vi "Line Garage.vi"() -> ()   [LabVIEW 2017]
uses:
  <vilib>/Instr/_visa.llb/VISA Configure Serial Port (Instr).vi
  <vilib>/Utility/inputDevices.llb/keyboardAcquire.vi
panel:
  in  "Tab Control":T1(tab)
  in  "COM PORT":refnum<visa-resource-name>
  in  "Cancel Button":bool
  in  "increment":dbl
  in  "TURBINE":dbl
  out "Waveform Chart":cluster{i32, i32}(graph)
  out "RIGHT RPM":dbl
  out "LEFT RPM":dbl
  in  "RPM":bool
  out "Right Power":dbl
  out "Left Power":dbl
  out "Monitor":string
  in  "Right Motor":dbl
  in  "Left Motor":dbl
  out "Right Meter":dbl(knob) scale=-1000.0..1000.0
  out "Left Meter":dbl(knob) scale=-1000.0..1000.0
  out "RPM Graph":cluster{i32, i32}(graph)
  in  "Update":bool
  out "Right Count":dbl
  out "Left Count":dbl
  out "Sen 15":dbl
  out "Sensor 15":dbl(slide) scale=0.0..4095.0
  out "Sen 14":dbl
  out "Sensor 14":dbl(slide) scale=0.0..4095.0
  out "Sen 12":dbl
  out "Sen 11":dbl
  out "Sen 10":dbl
  out "Sen 9":dbl
  out "Sen 8":dbl
  out "Sen 7":dbl
  out "Sen 6":dbl
  out "Sen 5":dbl
  out "Sen 4":dbl
  out "Sen 3":dbl
  out "Sen 2":dbl
  out "Sen 1":dbl
  out "Sen 0":dbl
  out "Sensor 12":dbl(slide) scale=0.0..4095.0
  out "Sensor 10":dbl(slide) scale=0.0..4095.0
  out "Sensor 9":dbl(slide) scale=0.0..4095.0
  out "Sensor 8":dbl(slide) scale=0.0..4095.0
  out "Sensor 7":dbl(slide) scale=0.0..4095.0
  out "Sensor 6":dbl(slide) scale=0.0..4095.0
  out "Sensor 5":dbl(slide) scale=0.0..4095.0
  out "Sensor 4":dbl(slide) scale=0.0..4095.0
  out "Sensor 3":dbl(slide) scale=0.0..4095.0
  out "Sensor 2":dbl(slide) scale=0.0..4095.0
  out "Sensor 1":dbl(slide) scale=0.0..4095.0
  out "Sensor 0":dbl(slide) scale=0.0..4095.0
  out "Sensor 11":dbl(slide) scale=0.0..4095.0
  in  "Update Sensors":bool
  out "Sensor 13":dbl(slide) scale=0.0..4095.0
  out "Sen 13":dbl
  in  "Read Calibration":bool
  in  "Save Calibration EEPROM":bool
  out "Max 14":dbl
  out "Min 14":dbl
  out "SenM 14":dbl
  out "SensorM 14":dbl(slide) scale=0.0..1000.0
  out "Max 13":dbl
  out "Min 13":dbl
  out "SenM 13":dbl
  out "SensorM 13":dbl(slide) scale=0.0..1000.0
  out "Max 12":dbl
  out "Max 11":dbl
  out "Max 10":dbl
  out "Max 9":dbl
  out "Max 8":dbl
  out "Max 7":dbl
  out "Max 6":dbl
  out "Max 5":dbl
  out "Max 4":dbl
  out "Max 3":dbl
  out "Max 2":dbl
  out "Max 1":dbl
  out "Max 0":dbl
  out "Min 12":dbl
  out "Min 11":dbl
  out "Min 10":dbl
  out "Min 9":dbl
  out "Min 8":dbl
  out "Min 7":dbl
  out "Min 6":dbl
  out "Min 5":dbl
  out "Min 4":dbl
  out "Min 3":dbl
  out "Min 2":dbl
  out "Min 1":dbl
  out "Min 0":dbl
  out "SenM 12":dbl
  out "SenM 11":dbl
  out "SenM 10":dbl
  out "SenM 9":dbl
  out "SenM 8":dbl
  out "SenM 7":dbl
  out "SenM 6":dbl
  out "SenM 5":dbl
  out "SenM 4":dbl
  out "SenM 3":dbl
  out "SenM 2":dbl
  out "SenM 1":dbl
  out "SenM 0":dbl
  out "SensorM 12":dbl(slide) scale=0.0..1000.0
  out "SensorM 10":dbl(slide) scale=0.0..1000.0
  out "SensorM 9":dbl(slide) scale=0.0..1000.0
  out "SensorM 8":dbl(slide) scale=0.0..1000.0
  out "SensorM 7":dbl(slide) scale=0.0..1000.0
  out "SensorM 6":dbl(slide) scale=0.0..1000.0
  out "SensorM  5":dbl(slide) scale=0.0..1000.0
  out "SensorM 4":dbl(slide) scale=0.0..1000.0
  out "SensorM 3":dbl(slide) scale=0.0..1000.0
  out "SensorM 2":dbl(slide) scale=0.0..1000.0
  out "SensorM 1":dbl(slide) scale=0.0..1000.0
  out "SensorM 0":dbl(slide) scale=0.0..1000.0
  out "SensorM 11":dbl(slide) scale=0.0..1000.0
  in  "Update Sensors 2":bool
  out "SensorM 15":dbl(slide) scale=0.0..1000.0
  out "SenM 15":dbl
  out "Min 15":dbl
  out "Max 15":dbl
  out "Position":dbl
  in  "Graph":bool
  out "Position":cluster{i32, i32}(graph)
  in  "Up Turbine":bool
  in  "Read Values":bool
  in  "Read EEPROM":bool
  in  "Save EEPROM":bool
  in  "Up Max":bool
  in  "Up Min":bool
  in  "Max Rang":dbl
  in  "Min Rang":dbl
  in  "Turbine Speed":dbl
  in  "Max In_1":dbl
  in  "Max D_1":dbl
  in  "Up MainSpeed":bool
  in  "Main Speed":dbl
  in  "Up Button1":bool
  in  "Kd_1":dbl
  in  "Ki_1":dbl
  in  "sample Time_1":dbl
  in  "SetPoint_1":dbl
  in  "Kp_1":dbl
  in  "Kp_2":dbl
  in  "SetPoint_2":dbl
  in  "sample Time_2":dbl
  in  "Ki_2":dbl
  in  "Kd_2":dbl
  in  "Up Button 2":bool
  in  "Max D_2":dbl
  in  "Max In_2":dbl
  in  "Max In_3":dbl
  in  "Max D_3":dbl
  in  "Up Button 3":bool
  in  "Kd_3":dbl
  in  "Ki_3":dbl
  in  "sample Time_3":dbl
  in  "SetPoint_3":dbl
  in  "Kp_3":dbl
  # "RIGHT"
  # "Motors"
  # "LEFT"
  # "Encoders Counts"
  # "LATERAL_PID"
  # "Turbine_PID"
  # "Central"
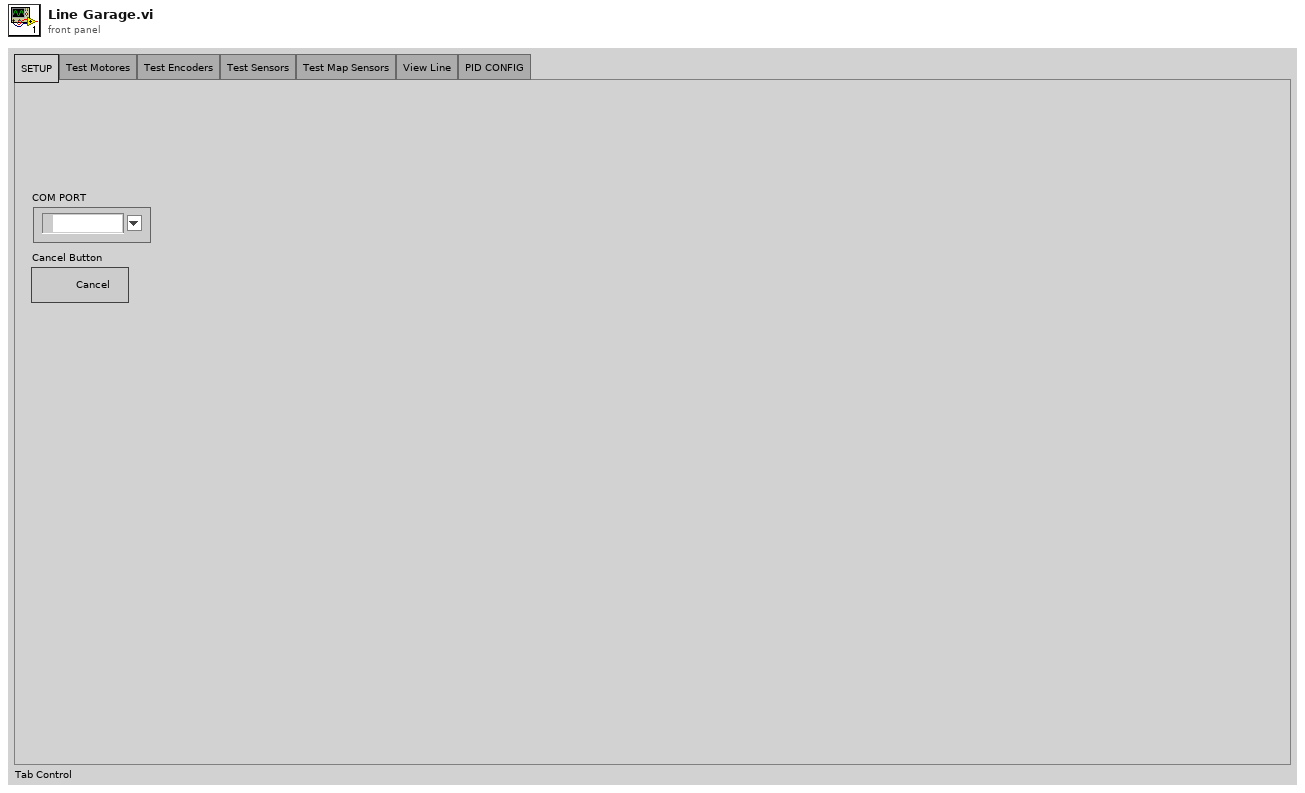
[diagram p1: front panel]
types:
  T1 = enum32{"SETUP", "Test Motores", "Test Encoders", "Test Sensors", "Test Map Sensors", "View Line", "PID CONFIG"}
  T2 = enum16{"0", "1", "2", "3", "4", "5", "6", "7", "8", "9", "A", "B", "C", "D", "E", "F", "G", "H", "I", "J", "K", "L", "M", "N", "O", "P", "Q", "R", "S", "T", "U", "V", "W", "X", "Y", "Z", "F1", "F2", "F3", "F4", "F5", "F6", "F7", "F8", "F9", "F10", "F11", "F12", "F13", "F14", "F15", "ADD", "BACK", "BACKSLASH", "CAPITAL", "COMMA", "DECIMAL", "DELETE", "DIVIDE", "DOWN", "END", "EQUALS", "ESCAPE", "GRAVE (`)", "HOME", "INSERT", "LBRACKET", "LCONTROL", "LEFT", "L ALT", "LSHIFT", "LWIN", "MINUS", "MULTIPLY", "NEXT", "NUMLOCK", "NUMPAD_0", "NUMPAD_1", "NUMPAD_2", "NUMPAD_3", "NUMPAD_4", "NUMPAD_5", "NUMPAD_6", "NUMPAD_7", "NUMPAD_8", "NUMPAD_9", "PAUSE", "PERIOD", "PRIOR (PG UP)", "RBRACKET", "RCONTROL", "RETURN", "RIGHT", "R ALT", "RSHIFT", "RWIN", "SCROLL", "SEMICOLON", "SLASH", "SPACE", "SUBTRACT", "TAB", "UP", "ENTER (num pad)", "' (quote)"}[]
  T3 = enum16{"0", "1", "2", "3", "4", "5", "6", "7", "8", "9", "A", "B", "C", "D", "E", "F", "G", "H", "I", "J", "K", "L", "M", "N", "O", "P", "Q", "R", "S", "T", "U", "V", "W", "X", "Y", "Z", "F1", "F2", "F3", "F4", "F5", "F6", "F7", "F8", "F9", "F10", "F11", "F12", "F13", "F14", "F15", "ADD", "BACK", "BACKSLASH", "CAPITAL", "COMMA", "DECIMAL", "DELETE", "DIVIDE", "DOWN", "END", "EQUALS", "ESCAPE", "GRAVE (`)", "HOME", "INSERT", "LBRACKET", "LCONTROL", "LEFT", "L ALT", "LSHIFT", "LWIN", "MINUS", "MULTIPLY", "NEXT", "NUMLOCK", "NUMPAD_0", "NUMPAD_1", "NUMPAD_2", "NUMPAD_3", "NUMPAD_4", "NUMPAD_5", "NUMPAD_6", "NUMPAD_7", "NUMPAD_8", "NUMPAD_9", "PAUSE", "PERIOD", "PRIOR (PG UP)", "RBRACKET", "RCONTROL", "RETURN", "RIGHT", "R ALT", "RSHIFT", "RWIN", "SCROLL", "SEMICOLON", "SLASH", "SPACE", "SUBTRACT", "TAB", "UP", "ENTER (num pad)", "' (quote)"}
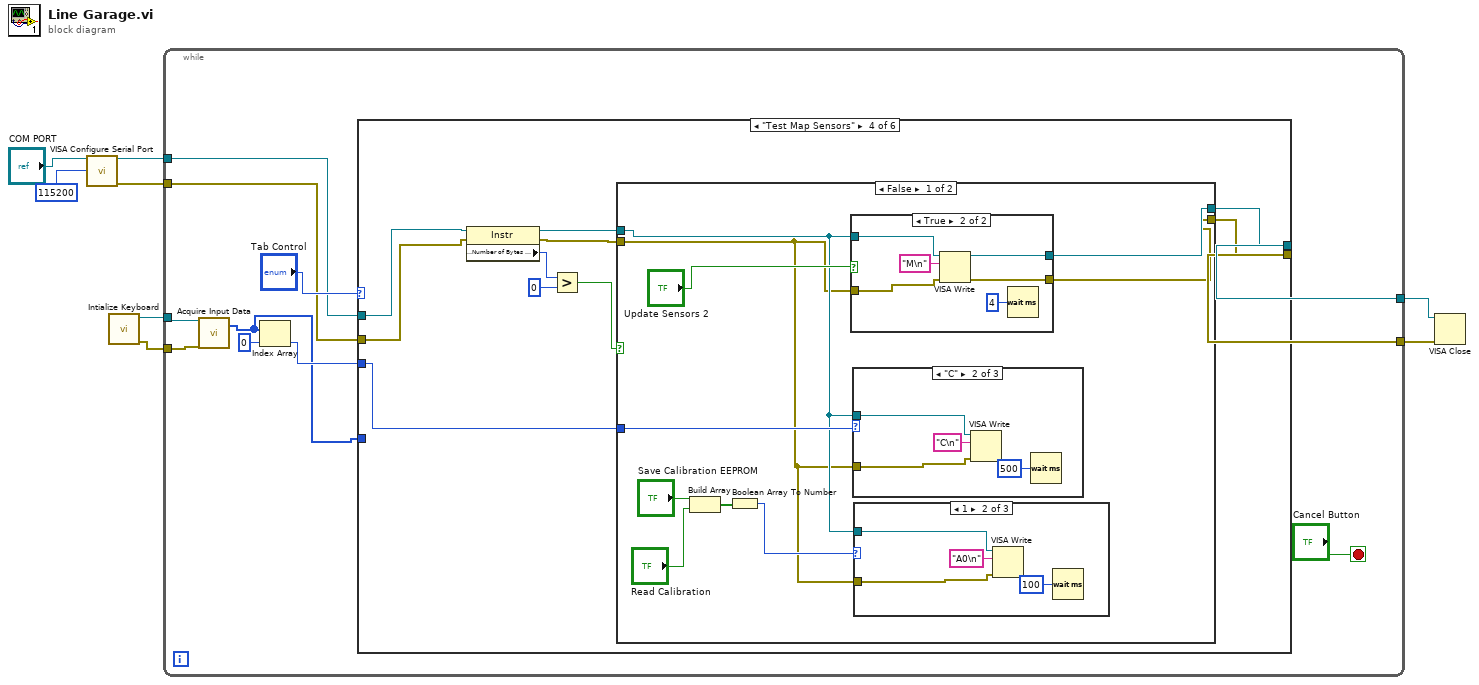
[diagram p0: block diagram]
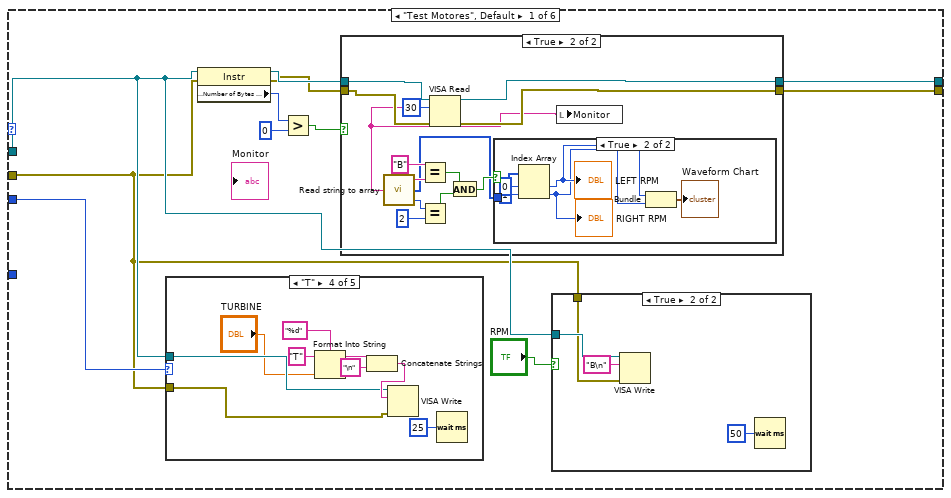
[diagram p2: hidden frame]
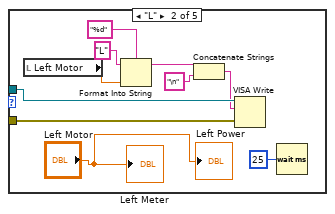
[diagram p7: hidden frame]
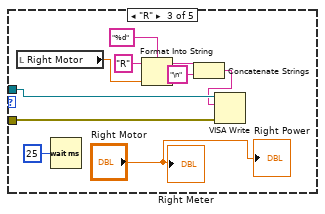
[diagram p8: hidden frame]
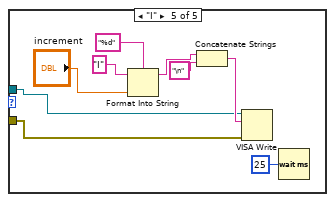
[diagram p9: hidden frame]
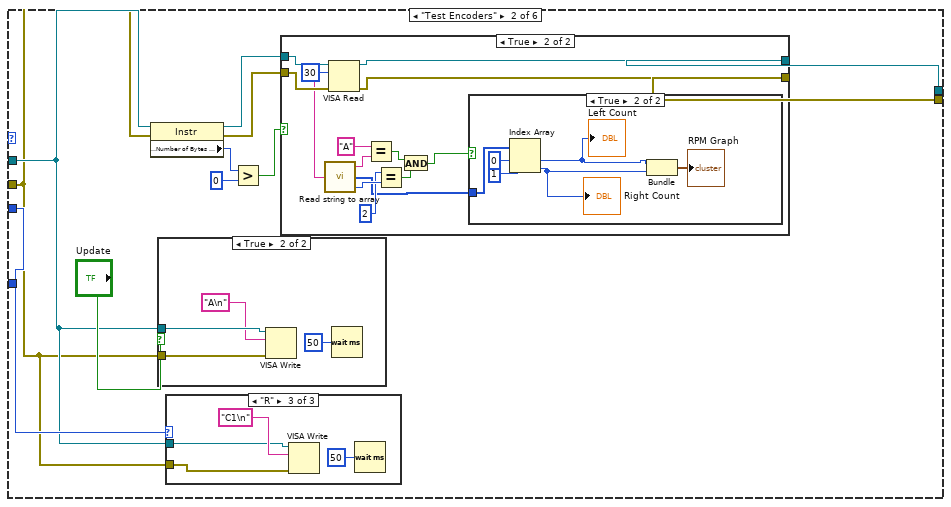
[diagram p10: hidden frame]
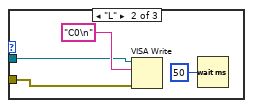
[diagram p12: hidden frame]
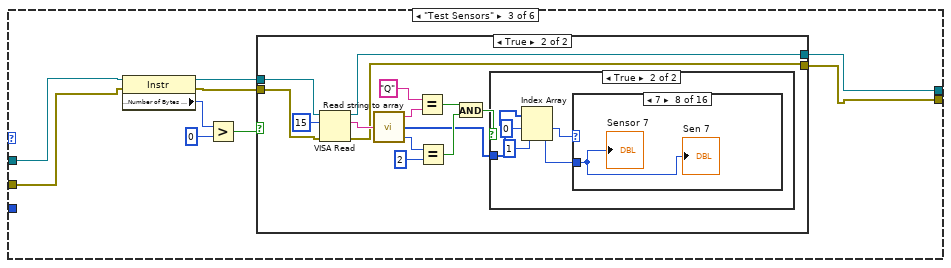
[diagram p16: hidden frame]
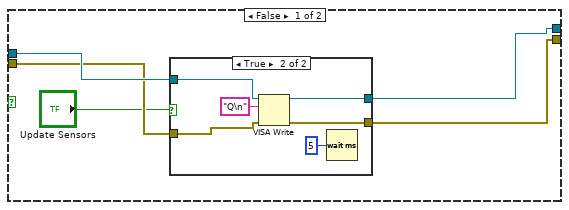
[diagram p17: hidden frame]
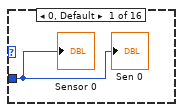
[diagram p20: hidden frame]
diagram:
  n1 = call-poly "VISA Configure Serial Port"("VISA resource name"="COM PORT", "baud rate (9600)"=u32 115200) -> ("VISA resource name out"=w4:refnum<visa-resource-name>, "error out"=w3:errorcluster)  [unwired: 12 in]
  n2 = call <vilib>:"Intialize Keyboard.vi"() -> ("error out"=w7:errorcluster, "device ID"=w8:refnum<k1>)  [unwired: 10 in]
  n3 = while {
    tunnel: w8 -> [w18]
    tunnel: w7 -> [w17]
    tunnel: w4 -> [w13]
    tunnel: w3 -> [w12]
    tunnel: [w11] -> w2
    tunnel: [w10] -> w1
    stop <- "Cancel Button" stop-if-true
    n4 = call-poly <vilib>:"Acquire Input Data.vi"("device ID"=w18, "error in (no error)"=w17) -> ("keys pressed"=w9:T2)  [unwired: 15 in, 2 out]
    n5 = Index Array(array=w9, index=0) -> (element=w14:T3)
    n6 = case shown="\"Test Map Sensors\"" "Tab Control" {
      tunnel: w14 -> [w30 w97 _ w197 _ w365]
      tunnel: w13 -> [w21 w96 w141 w204 w332 w374]
      tunnel: w12 -> [w20 w95 w140 w203 w331 w373]
      tunnel: [w25 w100 w142 w198 w324 w367] -> w11
      tunnel: [w23 w98 w143 w199 w325 w366] -> w10
      tunnel: w9 -> [_ _ _ _ _ _]
      frame "Test Motores", Default {
        n7 = case shown="\"T\"" w30 {
          tunnel: w21 -> [_ w66 w75 w78 w88]
          tunnel: w20 -> [_ w65 w74 w79 w87]
          frame "0", Default {
          }
          frame "L" {
            n8 = local read "Left Motor"() -> (w61:dbl)
            n9 = Format Into String(format string="%d", initial string="L", w61) -> (resulting string=w60:string)  [unwired: 1 in, 1 out]
            n10 = Concatenate Strings(w60, "\n" ("string")) -> (w58:string)
            n11 = VISA Write(VISA resource name=w66, write buffer=w58, error in (no error)=w65) -> ()  [unwired: 3 out]
            n12 = Wait (ms)(milliseconds to wait=u32 25) -> ()  [unwired: 1 out]
            "Left Meter" <- "Left Motor"
            "Left Power" <- "Left Motor"
          }
          frame "R" {
            n13 = local read "Right Motor"() -> (w71:dbl)
            n14 = Wait (ms)(milliseconds to wait=u32 25) -> ()  [unwired: 1 out]
            n15 = Format Into String(format string="%d", initial string="R", w71) -> (resulting string=w69:string)  [unwired: 1 in, 1 out]
            n16 = Concatenate Strings(w69, "\n" ("string")) -> (w70:string)
            n17 = VISA Write(VISA resource name=w75, write buffer=w70, error in (no error)=w74) -> ()  [unwired: 3 out]
            "Right Meter" <- "Right Motor"
            "Right Power" <- "Right Motor"
          }
          frame "T" {
            n18 = Format Into String(format string="%d", initial string="T", "TURBINE") -> (resulting string=w81:string)  [unwired: 1 in, 1 out]
            n19 = Concatenate Strings(w81, "\n" ("string")) -> (w82:string)
            n20 = VISA Write(VISA resource name=w78, write buffer=w82, error in (no error)=w79) -> ()  [unwired: 3 out]
            n21 = Wait (ms)(milliseconds to wait=u32 25) -> ()  [unwired: 1 out]
          }
          frame "I" {
            n22 = Format Into String(format string="%d", initial string="I", "increment") -> (resulting string=w91:string)  [unwired: 1 in, 1 out]
            n23 = Concatenate Strings(w91, "\n") -> (w89:string)
            n24 = VISA Write(VISA resource name=w88, write buffer=w89, error in (no error)=w87) -> ()  [unwired: 3 out]
            n25 = Wait (ms)(milliseconds to wait=u32 25) -> ()  [unwired: 1 out]
          }
        }
        n26 = property class="Instr"(reference=w21, error in=w20) -> (reference out=w26:refnum<visa-resource-name>, error out=w24:errorcluster, "Serial Settings:Number of Bytes at Serial Port"=w29:u32)
        n27 = Greater?(x=w29, y=u32 0) -> (0:w27:bool)
        n28 = case shown="True" w27 {
          tunnel: [w36 w48] -> w25
          tunnel: w26 -> [w36 w50]
          tunnel: w24 -> [w35 w49]
          tunnel: [w35 w47] -> w23
          frame False {
          }
          frame True {
            n29 = VISA Read(VISA resource name=w50, byte count=u32 30, error in (no error)=w49) -> (VISA resource name out=w48:refnum<visa-resource-name>, read buffer=w45:string, error out=w47:errorcluster)  [unwired: 1 out]
            n30 = call "Read string to array.vi"("String"=w45) -> ("size(s)"=w40:i32, "Array"=w37:i32[], "caracter"=w44:string)  [unwired: 2 in]
            n31 = Equal?(x="B", y=w44) -> (x = y?=w42:bool)
            n32 = Equal?(x=w40, y=2) -> (x = y?=w41:bool)
            n33 = And(x=w42, y=w41) -> (x .and. y?=w38:bool)
            n34 = case shown="True" w38 {
              tunnel: w37 -> [_ w56]
              frame False {
              }
              frame True {
                n35 = Index Array(array=w56, index #1=0 ("index"), index #2=1 ("index")) -> (element #1=w53:i32, element #2=w52:i32)
                "LEFT RPM" <- w53
                "RIGHT RPM" <- w52
                n36 = Bundle(w53, w52) -> (→"Waveform Chart":cluster{i32, i32})  [unwired: 1 in]
              }
            }
            n37 = local write "Monitor"(w45) -> ()
          }
        }
        n38 = case shown="True" "RPM" {
          tunnel: w21 -> [_ w34]
          tunnel: w20 -> [_ w33]
          frame False {
          }
          frame True {
            n39 = VISA Write(VISA resource name=w34, write buffer="B\n", error in (no error)=w33) -> ()  [unwired: 3 out]
            n40 = Wait (ms)(milliseconds to wait=u32 50) -> ()  [unwired: 1 out]
          }
        }
      }
      frame "Test Encoders" {
        n41 = property class="Instr"(reference=w96, error in=w95) -> (reference out=w101:refnum<visa-resource-name>, error out=w99:errorcluster, "Serial Settings:Number of Bytes at Serial Port"=w104:u32)
        n42 = case shown="True" "Update" {
          tunnel: w96 -> [_ w138]
          tunnel: w95 -> [_ w137]
          frame False {
          }
          frame True {
            n43 = VISA Write(VISA resource name=w138, write buffer="A\n", error in (no error)=w137) -> ()  [unwired: 3 out]
            n44 = Wait (ms)(milliseconds to wait=u32 50) -> ()  [unwired: 1 out]
          }
        }
        n45 = case shown="\"R\"" w97 {
          tunnel: w96 -> [_ w107 w111]
          tunnel: w95 -> [_ w106 w110]
          frame "0", Default {
          }
          frame "L" {
            n46 = VISA Write(VISA resource name=w107, write buffer="C0\n", error in (no error)=w106) -> ()  [unwired: 3 out]
            n47 = Wait (ms)(milliseconds to wait=u32 50) -> ()  [unwired: 1 out]
          }
          frame "R" {
            n48 = VISA Write(VISA resource name=w111, write buffer="C1\n", error in (no error)=w110) -> ()  [unwired: 3 out]
            n49 = Wait (ms)(milliseconds to wait=u32 50) -> ()  [unwired: 1 out]
          }
        }
        n50 = Greater?(x=w104, y=u32 0) -> (0:w102:bool)
        n51 = case shown="True" w102 {
          tunnel: [w115 w126] -> w100
          tunnel: w101 -> [w115 w129]
          tunnel: [w114 w125] -> w98
          tunnel: w99 -> [w114 w128]
          frame False {
          }
          frame True {
            n52 = VISA Read(VISA resource name=w129, byte count=u32 30, error in (no error)=w128) -> (VISA resource name out=w126:refnum<visa-resource-name>, read buffer=w124:string, error out=w125:errorcluster)  [unwired: 1 out]
            n53 = call "Read string to array.vi"("String"=w124) -> ("size(s)"=w120:i32, "Array"=w116:i32[], "caracter"=w123:string)  [unwired: 2 in]
            n54 = Equal?(x="A", y=w123) -> (x = y?=w121:bool)
            n55 = Equal?(x=2, y=w120) -> (x = y?=w118:bool)
            n56 = And(x=w121, y=w118) -> (x .and. y?=w117:bool)
            n57 = case shown="True" w117 {
              tunnel: w116 -> [_ w135]
              frame False {
              }
              frame True {
                n58 = Index Array(array=w135, index #1=0 ("index"), index #2=1 ("index")) -> (element #1=w132:i32, element #2=w130:i32)
                "Right Count" <- w130
                "Left Count" <- w132
                n59 = Bundle(w132, w130) -> (→"RPM Graph":cluster{i32, i32})  [unwired: 1 in]
              }
            }
          }
        }
      }
      frame "Test Sensors" {
        n60 = property class="Instr"(reference=w141, error in=w140) -> (reference out=w145:refnum<visa-resource-name>, error out=w144:errorcluster, "Serial Settings:Number of Bytes at Serial Port"=w148:u32)
        n61 = Greater?(x=w148, y=u32 0) -> (0:w146:bool)
        n62 = case shown="True" w146 {
          tunnel: w145 -> [w153 w175]
          tunnel: w144 -> [w152 w174]
          tunnel: [w150 w163] -> w142
          tunnel: [w149 w162] -> w143
          frame False {
            n63 = case shown="True" "Update Sensors" {
              tunnel: w153 -> [w155 w160]
              tunnel: w152 -> [w154 w159]
              tunnel: [w155 w158] -> w150
              tunnel: [w154 w157] -> w149
              frame False {
              }
              frame True {
                n64 = VISA Write(VISA resource name=w160, write buffer="Q\n", error in (no error)=w159) -> (VISA resource name out=w158:refnum<visa-resource-name>, error out=w157:errorcluster)  [unwired: 1 out]
                n65 = Wait (ms)(milliseconds to wait=u32 5) -> ()  [unwired: 1 out]
              }
            }
          }
          frame True {
            n66 = VISA Read(VISA resource name=w175, byte count=u32 15, error in (no error)=w174) -> (VISA resource name out=w163:refnum<visa-resource-name>, read buffer=w172:string, error out=w162:errorcluster)  [unwired: 1 out]
            n67 = call "Read string to array.vi"("String"=w172) -> ("size(s)"=w169:i32, "Array"=w164:i32[], "caracter"=w171:string)  [unwired: 2 in]
            n68 = Equal?(x="Q", y=w171) -> (x = y?=w167:bool)
            n69 = Equal?(x=w169, y=2) -> (x = y?=w166:bool)
            n70 = And(x=w167, y=w166) -> (x .and. y?=w165:bool)
            n71 = case shown="True" w165 {
              tunnel: w164 -> [_ w180]
              frame False {
              }
              frame True {
                n72 = Index Array(array=w180, index #1=0 ("index"), index #2=1 ("index")) -> (element #1=w177:i32, element #2=w176:i32)
                n73 = case shown="7" w177 {
                  tunnel: w176 -> [w181 w182 w183 w184 w185 w186 w187 w188 w189 w190 w191 w192 w193 w194 w195 w196]
                  frame 0, Default {
                    "Sensor 0" <- w181
                    "Sen 0" <- w181
                  }
                  frame 1 {
                    "Sensor 1" <- w182
                    "Sen 1" <- w182
                  }
                  frame 2 {
                    "Sen 2" <- w183
                    "Sensor 2" <- w183
                  }
                  frame 3 {
                    "Sensor 3" <- w184
                    "Sen 3" <- w184
                  }
                  frame 4 {
                    "Sensor 4" <- w185
                    "Sen 4" <- w185
                  }
                  frame 5 {
                    "Sen 5" <- w186
                    "Sensor 5" <- w186
                  }
                  frame 6 {
                    "Sensor 6" <- w187
                    "Sen 6" <- w187
                  }
                  frame 7 {
                    "Sensor 7" <- w188
                    "Sen 7" <- w188
                  }
                  frame 8 {
                    "Sensor 8" <- w189
                    "Sen 8" <- w189
                  }
                  frame 9 {
                    "Sensor 9" <- w190
                    "Sen 9" <- w190
                  }
                  frame 10 {
                    "Sensor 10" <- w191
                    "Sen 10" <- w191
                  }
                  frame 11 {
                    "Sensor 11" <- w192
                    "Sen 11" <- w192
                  }
                  frame 12 {
                    "Sen 12" <- w193
                    "Sensor 12" <- w193
                  }
                  frame 13 {
                    "Sen 13" <- w194
                    "Sensor 13" <- w194
                  }
                  frame 14 {
                    "Sensor 14" <- w195
                    "Sen 14" <- w195
                  }
                  frame 15 {
                    "Sensor 15" <- w196
                    "Sen 15" <- w196
                  }
                }
              }
            }
          }
        }
      }
      frame "Test Map Sensors" {
        n74 = property class="Instr"(reference=w204, error in=w203) -> (reference out=w201:refnum<visa-resource-name>, error out=w200:errorcluster, "Serial Settings:Number of Bytes at Serial Port"=w206:u32)
        n75 = Greater?(x=w206, y=u32 0) -> (0:w202:bool)
        n76 = case shown="False" w202 {
          tunnel: w201 -> [w208 w259]
          tunnel: w200 -> [w207 w258]
          tunnel: [w215 w253] -> w198
          tunnel: [w214 w252] -> w199
          tunnel: w197 -> [w213 _]
          frame False {
            n77 = Build Array("Save Calibration EEPROM", "Read Calibration") -> (w210:bool[])
            n78 = Boolean Array To Number(Boolean array=w210) -> (number=w209:u32)
            n79 = case shown="True" "Update Sensors 2" {
              tunnel: w208 -> [w234 w239]
              tunnel: w207 -> [w233 w238]
              tunnel: [w234 w237] -> w215
              tunnel: [w233 w236] -> w214
              frame False {
              }
              frame True {
                n80 = VISA Write(VISA resource name=w239, write buffer="M\n", error in (no error)=w238) -> (VISA resource name out=w237:refnum<visa-resource-name>, error out=w236:errorcluster)  [unwired: 1 out]
                n81 = Wait (ms)(milliseconds to wait=u32 4) -> ()  [unwired: 1 out]
              }
            }
            n82 = case shown="\"C\"" w213 {
              tunnel: w208 -> [_ w227 w230]
              tunnel: w207 -> [_ w226 w229]
              frame "0", Default {
              }
              frame "C" {
                n83 = VISA Write(VISA resource name=w227, write buffer="C\n", error in (no error)=w226) -> ()  [unwired: 3 out]
                n84 = Wait (ms)(milliseconds to wait=u32 500) -> ()  [unwired: 1 out]
              }
              frame "G" {
                n85 = VISA Write(VISA resource name=w230, write buffer="G\n", error in (no error)=w229) -> ()  [unwired: 3 out]
                n86 = Wait (ms)(milliseconds to wait=u32 500) -> ()  [unwired: 1 out]
              }
            }
            n87 = case shown="1" w209 {
              tunnel: w208 -> [_ w218 w221]
              tunnel: w207 -> [_ w217 w222]
              frame 0, Default {
              }
              frame 1 {
                n88 = VISA Write(VISA resource name=w218, write buffer="A0\n", error in (no error)=w217) -> ()  [unwired: 3 out]
                n89 = Wait (ms)(milliseconds to wait=u32 100) -> ()  [unwired: 1 out]
              }
              frame 2 {
                n90 = VISA Write(VISA resource name=w221, write buffer="B0\n", error in (no error)=w222) -> ()  [unwired: 3 out]
                n91 = Wait (ms)(milliseconds to wait=u32 100) -> ()  [unwired: 1 out]
              }
            }
          }
          frame True {
            n92 = VISA Read(VISA resource name=w259, byte count=u32 15, error in (no error)=w258) -> (VISA resource name out=w253:refnum<visa-resource-name>, read buffer=w247:string, error out=w252:errorcluster)  [unwired: 1 out]
            n93 = call "Read string to array.vi"("String"=w247) -> ("size(s)"=w251:i32, "Array"=w242:i32[], "caracter"=w241:string)  [unwired: 2 in]
            n94 = Equal?(x=w241, y="U") -> (x = y?=w248:bool)
            n95 = Equal?(x="M", y=w241) -> (x = y?=w255:bool)
            n96 = Equal?(x=w251, y=2) -> (x = y?=w245:bool)
            n97 = And(x=w248, y=w245) -> (x .and. y?=w249:bool)
            n98 = case shown="True" w249 {
              tunnel: w242 -> [_ w286]
              frame False {
              }
              frame True {
                n99 = Index Array(array=w286, index #1=0 ("index"), index #2=1 ("index")) -> (element #1=w283:i32, element #2=w282:i32)
                n100 = case shown="15" w283 {
                  tunnel: w282 -> [w287 w288 w289 w290 w291 w292 w293 w294 w295 w296 w297 w298 w299 w300 w301 w302]
                  frame 0, Default {
                    "Max 0" <- w287
                  }
                  frame 1 {
                    "Max 1" <- w288
                  }
                  frame 2 {
                    "Max 2" <- w289
                  }
                  frame 3 {
                    "Max 3" <- w290
                  }
                  frame 4 {
                    "Max 4" <- w291
                  }
                  frame 5 {
                    "Max 5" <- w292
                  }
                  frame 6 {
                    "Max 6" <- w293
                  }
                  frame 7 {
                    "Max 7" <- w294
                  }
                  frame 8 {
                    "Max 8" <- w295
                  }
                  frame 9 {
                    "Max 9" <- w296
                  }
                  frame 10 {
                    "Max 10" <- w297
                  }
                  frame 11 {
                    "Max 11" <- w298
                  }
                  frame 12 {
                    "Max 12" <- w299
                  }
                  frame 13 {
                    "Max 13" <- w300
                  }
                  frame 14 {
                    "Max 14" <- w301
                  }
                  frame 15 {
                    "Max 15" <- w302
                  }
                }
              }
            }
            n101 = And(x=w255, y=w245) -> (x .and. y?=w254:bool)
            n102 = case shown="True" w254 {
              tunnel: w242 -> [_ w307]
              frame False {
              }
              frame True {
                n103 = Index Array(array=w307, index #1=0 ("index"), index #2=1 ("index")) -> (element #1=w304:i32, element #2=w303:i32)
                n104 = case shown="15" w304 {
                  tunnel: w303 -> [w308 w309 w310 w311 w312 w313 w314 w315 w316 w317 w318 w319 w320 w321 w322 w323]
                  frame 0, Default {
                    "SenM 0" <- w308
                    "SensorM 0" <- w308
                  }
                  frame 1 {
                    "SenM 1" <- w309
                    "SensorM 1" <- w309
                  }
                  frame 2 {
                    "SensorM 2" <- w310
                    "SenM 2" <- w310
                  }
                  frame 3 {
                    "SensorM 3" <- w311
                    "SenM 3" <- w311
                  }
                  frame 4 {
                    "SensorM 4" <- w312
                    "SenM 4" <- w312
                  }
                  frame 5 {
                    "SensorM  5" <- w313
                    "SenM 5" <- w313
                  }
                  frame 6 {
                    "SensorM 6" <- w314
                    "SenM 6" <- w314
                  }
                  frame 7 {
                    "SensorM 7" <- w315
                    "SenM 7" <- w315
                  }
                  frame 8 {
                    "SensorM 8" <- w316
                    "SenM 8" <- w316
                  }
                  frame 9 {
                    "SenM 9" <- w317
                    "SensorM 9" <- w317
                  }
                  frame 10 {
                    "SensorM 10" <- w318
                    "SenM 10" <- w318
                  }
                  frame 11 {
                    "SensorM 11" <- w319
                    "SenM 11" <- w319
                  }
                  frame 12 {
                    "SenM 12" <- w320
                    "SensorM 12" <- w320
                  }
                  frame 13 {
                    "SenM 13" <- w321
                    "SensorM 13" <- w321
                  }
                  frame 14 {
                    "SensorM 14" <- w322
                    "SenM 14" <- w322
                  }
                  frame 15 {
                    "SensorM 15" <- w323
                    "SenM 15" <- w323
                  }
                }
              }
            }
            n105 = Equal?(x=w241, y="L") -> (x = y?=w244:bool)
            n106 = And(x=w245, y=w244) -> (x .and. y?=w243:bool)
            n107 = case shown="True" w243 {
              tunnel: w242 -> [_ w265]
              frame False {
              }
              frame True {
                n108 = Index Array(array=w265, index #1=0 ("index"), index #2=1 ("index")) -> (element #1=w262:i32, element #2=w261:i32)
                n109 = case shown="15" w262 {
                  tunnel: w261 -> [w266 w267 w268 w269 w270 w271 w272 w273 w274 w275 w276 w277 w278 w279 w280 w281]
                  frame 0, Default {
                    "Min 0" <- w266
                  }
                  frame 1 {
                    "Min 1" <- w267
                  }
                  frame 2 {
                    "Min 2" <- w268
                  }
                  frame 3 {
                    "Min 3" <- w269
                  }
                  frame 4 {
                    "Min 4" <- w270
                  }
                  frame 5 {
                    "Min 5" <- w271
                  }
                  frame 6 {
                    "Min 6" <- w272
                  }
                  frame 7 {
                    "Min 7" <- w273
                  }
                  frame 8 {
                    "Min 8" <- w274
                  }
                  frame 9 {
                    "Min 9" <- w275
                  }
                  frame 10 {
                    "Min 10" <- w276
                  }
                  frame 11 {
                    "Min 11" <- w277
                  }
                  frame 12 {
                    "Min 12" <- w278
                  }
                  frame 13 {
                    "Min 13" <- w279
                  }
                  frame 14 {
                    "Min 14" <- w280
                  }
                  frame 15 {
                    "Min 15" <- w281
                  }
                }
              }
            }
          }
        }
      }
      frame "View Line" {
        n110 = property class="Instr"(reference=w332, error in=w331) -> (reference out=w327:refnum<visa-resource-name>, error out=w326:errorcluster, "Serial Settings:Number of Bytes at Serial Port"=w330:u32)
        n111 = Greater?(x=w330, y=u32 0) -> (0:w328:bool)
        n112 = case shown="False" w328 {
          tunnel: w327 -> [w336 w359]
          tunnel: w326 -> [w334 w358]
          tunnel: [w335 w353] -> w324
          tunnel: [w333 w352] -> w325
          frame False {
            n113 = case shown="True" "Graph" {
              tunnel: w336 -> [w339 w345]
              tunnel: [w339 w344] -> w335
              tunnel: w334 -> [w338 w341]
              tunnel: [w338 w340] -> w333
              frame False {
              }
              frame True {
                n114 = VISA Write(VISA resource name=w345, write buffer="P\n", error in (no error)=w341) -> (VISA resource name out=w344:refnum<visa-resource-name>, error out=w340:errorcluster)  [unwired: 1 out]
                n115 = Wait (ms)(milliseconds to wait=u32 25) -> ()  [unwired: 1 out]
              }
            }
          }
          frame True {
            n116 = VISA Read(VISA resource name=w359, byte count=u32 15, error in (no error)=w358) -> (VISA resource name out=w353:refnum<visa-resource-name>, read buffer=w356:string, error out=w352:errorcluster)  [unwired: 1 out]
            n117 = call "Read string to array.vi"("String"=w356) -> ("size(s)"=w355:i32, "Array"=w346:i32[], "caracter"=w351:string)  [unwired: 2 in]
            n118 = Equal?(x=w355, y=1) -> (x = y?=w348:bool)
            n119 = Equal?(x="P", y=w351) -> (x = y?=w349:bool)
            n120 = And(x=w349, y=w348) -> (x .and. y?=w347:bool)
            n121 = case shown="True" w347 {
              tunnel: w346 -> [_ w364]
              frame False {
              }
              frame True {
                n122 = Index Array(array=w364, index=0) -> (element=w361:i32)
                "Position" <- w361
                n123 = Bundle(w361, 7500) -> (→"Position":cluster{i32, i32})  [unwired: 1 in]
              }
            }
          }
        }
      }
      frame "PID CONFIG" {
        n124 = property class="Instr"(reference=w374, error in=w373) -> (reference out=w369:refnum<visa-resource-name>, error out=w368:errorcluster, "Serial Settings:Number of Bytes at Serial Port"=w372:u32)
        n125 = Greater?(x=w372, y=u32 0) -> (0:w370:bool)
        n126 = case shown="False" w370 {
          tunnel: w369 -> [w383 w460]
          tunnel: w368 -> [w382 w461]
          tunnel: [w380 w460] -> w367
          tunnel: [w379 w461] -> w366
          tunnel: w365 -> [_ w459]
          frame True {
            n127 = VISA Read(VISA resource name=w383, byte count=u32 60, error in (no error)=w382) -> (VISA resource name out=w380:refnum<visa-resource-name>, read buffer=w378:string, error out=w379:errorcluster)  [unwired: 1 out]
            n128 = call "Read string to array.vi"("String"=w378) -> ("size(s)"=w375:i32, "Array"=w376:i32[], "caracter"=w377:string)  [unwired: 2 in]
            n129 = case shown="\"E\"" w377 {
              tunnel: w376 -> [_ w384 w391 w398 w405 w412]
              tunnel: w375 -> [_ w387 w393 w400 w407 w415]
              frame "False", Default {
              }
              frame "S" {
                n130 = Equal?(x=w387, y=1) -> (x = y?=w385:bool)
                n131 = case shown="True" w385 {
                  tunnel: w384 -> [_ w390]
                  frame False {
                  }
                  frame True {
                    n132 = Index Array(array=w390, index=0) -> (element=w388:i32)
                    n133 = local write "Main Speed"(w388) -> ()
                  }
                }
              }
              frame "E" {
                n134 = Equal?(x=w393, y=1) -> (x = y?=w392:bool)
                n135 = case shown="True" w392 {
                  tunnel: w391 -> [_ w397]
                  frame False {
                  }
                  frame True {
                    n136 = Index Array(array=w397, index=0) -> (element=w395:i32)
                    n137 = local write "Min Rang"(w395) -> ()
                  }
                }
              }
              frame "D" {
                n138 = Equal?(x=w400, y=1) -> (x = y?=w399:bool)
                n139 = case shown="True" w399 {
                  tunnel: w398 -> [_ w404]
                  frame False {
                  }
                  frame True {
                    n140 = Index Array(array=w404, index=0) -> (element=w402:i32)
                    n141 = local write "Max Rang"(w402) -> ()
                  }
                }
              }
              frame "T" {
                n142 = Equal?(x=w407, y=1) -> (x = y?=w406:bool)
                n143 = case shown="True" w406 {
                  tunnel: w405 -> [_ w411]
                  frame False {
                  }
                  frame True {
                    n144 = Index Array(array=w411, index=0) -> (element=w409:i32)
                    n145 = local write "Turbine Speed"(w409) -> ()
                  }
                }
              }
              frame "U" {
                n146 = Equal?(x=w415, y=3) -> (x = y?=w413:bool)
                n147 = case shown="True" w413 {
                  tunnel: w412 -> [_ w422]
                  frame False {
                  }
                  frame True {
                    n148 = Index Array(array=w422, index #1=0 ("index"), index #2=1 ("index"), index #3=2 ("index")) -> (element #1=w420:i32, element #2=w418:i32, element #3=w416:i32)
                    n149 = case shown="0, Default" w420 {
                      tunnel: w418 -> [w424 w433 w442]
                      tunnel: w416 -> [w423 w432 w441]
                      frame 0, Default {
                        n150 = case shown="6" w424 {
                          tunnel: w423 -> [w425 w426 w427 w428 w429 w430 w431]
                          frame 0, Default {
                            n151 = local write "Kp_1"(w425) -> ()
                          }
                          frame 1 {
                            n152 = local write "Ki_1"(w426) -> ()
                          }
                          frame 2 {
                            n153 = local write "Kd_1"(w427) -> ()
                          }
                          frame 3 {
                            n154 = local write "sample Time_1"(w428) -> ()
                          }
                          frame 4 {
                            n155 = local write "SetPoint_1"(w429) -> ()
                          }
                          frame 5 {
                            n156 = local write "Max D_1"(w430) -> ()
                          }
                          frame 6 {
                            n157 = local write "Max In_1"(w431) -> ()
                          }
                        }
                      }
                      frame 1 {
                        n158 = case shown="6" w433 {
                          tunnel: w432 -> [w434 w435 w436 w437 w438 w439 w440]
                          frame 0, Default {
                            n159 = local write "Kp_2"(w434) -> ()
                          }
                          frame 1 {
                            n160 = local write "Ki_2"(w435) -> ()
                          }
                          frame 2 {
                            n161 = local write "Kd_2"(w436) -> ()
                          }
                          frame 3 {
                            n162 = local write "sample Time_2"(w437) -> ()
                          }
                          frame 4 {
                            n163 = local write "SetPoint_2"(w438) -> ()
                          }
                          frame 5 {
                            n164 = local write "Max D_2"(w439) -> ()
                          }
                          frame 6 {
                            n165 = local write "Max In_2"(w440) -> ()
                          }
                        }
                      }
                      frame 2 {
                        n166 = case shown="6" w442 {
                          tunnel: w441 -> [w443 w444 w445 w446 w447 w448 w449]
                          frame 0, Default {
                            n167 = local write "Kp_3"(w443) -> ()
                          }
                          frame 1 {
                            n168 = local write "Ki_3"(w444) -> ()
                          }
                          frame 2 {
                            n169 = local write "Kd_3"(w445) -> ()
                          }
                          frame 3 {
                            n170 = local write "sample Time_3"(w446) -> ()
                          }
                          frame 4 {
                            n171 = local write "SetPoint_3"(w447) -> ()
                          }
                          frame 5 {
                            n172 = local write "Max D_3"(w448) -> ()
                          }
                          frame 6 {
                            n173 = local write "Max In_3"(w449) -> ()
                          }
                        }
                      }
                    }
                  }
                }
              }
            }
          }
          frame False {
            n174 = Build Array("Up Button1", "Up MainSpeed", "Up Button 2", "Up Button 3", "Up Min", "Up Max", "Up Turbine", "Read EEPROM", "Save EEPROM", "Read Values") -> (w464:bool[])
            n175 = Boolean Array To Number(Boolean array=w464) -> (number=w463:u32)
            n176 = case shown="256" w463 {
              tunnel: "U" -> [_ w470 _ w498 w517 _ _ _ _ _ _]
              tunnel: w460 -> [_ w467 w490 w496 w516 w536 w545 w554 w564 w572 w580]
              tunnel: w461 -> [_ w466 w491 w495 w515 w537 w546 w553 w563 w573 w581]
              tunnel: w459 -> [_ _ _ _ _ _ _ _ _ _ _]
              frame 0, Default {
              }
              frame 1 {
                n177 = for {
                  N: 7 -> [_]
                  tunnel: w470 -> [w478]
                  tunnel: 0 -> [w477]
                  tunnel: w467 -> [w474]
                  tunnel: w466 -> [w473]
                  i -> [w471]
                  n178 = case shown="6" w471 {
                    tunnel: ["Kp_1" "Ki_1" "Kd_1" "sample Time_1" "SetPoint_1" "Max D_1" "Max In_1"] -> w476
                    frame 0, Default {
                    }
                    frame 1 {
                    }
                    frame 2 {
                    }
                    frame 3 {
                    }
                    frame 4 {
                    }
                    frame 5 {
                    }
                    frame 6 {
                    }
                  }
                  n179 = call "senPID.vi"("Numeric 3"=w476, "Numeric 2"=w471, "Numeric"=w477, "String"=w478) -> ("String 2"=w472:string)
                  n180 = Wait (ms)(milliseconds to wait=u32 20) -> ()  [unwired: 1 out]
                  n181 = VISA Write(VISA resource name=w474, write buffer=w472, error in (no error)=w473) -> ()  [unwired: 3 out]
                }
              }
              frame 2 {
                n182 = Format Into String(format string="%d", initial string="S", "Main Speed") -> (resulting string=w489:string)  [unwired: 1 in, 1 out]
                n183 = Concatenate Strings(w489, "\n" ("string")) -> (w487:string)
                n184 = VISA Write(VISA resource name=w490, write buffer=w487, error in (no error)=w491) -> ()  [unwired: 3 out]
                n185 = Wait (ms)(milliseconds to wait=u32 10) -> ()  [unwired: 1 out]
              }
              frame 4 {
                n186 = for {
                  N: 8 -> [_]
                  tunnel: w498 -> [w507]
                  tunnel: 1 -> [w506]
                  tunnel: w496 -> [w501]
                  tunnel: w495 -> [w500]
                  i -> [w505]
                  n187 = case shown="5" w505 {
                    tunnel: ["Kp_2" "Ki_2" "Kd_2" "sample Time_2" "SetPoint_2" "Max D_2" "Max In_2"] -> w504
                    frame 0, Default {
                    }
                    frame 1 {
                    }
                    frame 2 {
                    }
                    frame 3 {
                    }
                    frame 4 {
                    }
                    frame 5 {
                    }
                    frame 6 {
                    }
                  }
                  n188 = call "senPID.vi"("Numeric 3"=w504, "Numeric 2"=w505, "Numeric"=w506, "String"=w507) -> ("String 2"=w502:string)
                  n189 = Wait (ms)(milliseconds to wait=u32 20) -> ()  [unwired: 1 out]
                  n190 = VISA Write(VISA resource name=w501, write buffer=w502, error in (no error)=w500) -> ()  [unwired: 3 out]
                }
              }
              frame 8 {
                n191 = for {
                  N: 8 -> [_]
                  tunnel: 2 -> [w524]
                  tunnel: w517 -> [w525]
                  tunnel: w516 -> [w521]
                  tunnel: w515 -> [w520]
                  i -> [w523]
                  n192 = case shown="6" w523 {
                    tunnel: ["Kp_3" "Ki_3" "Kd_3" "sample Time_3" "SetPoint_3" "Max D_3" "Max In_3"] -> w522
                    frame 0, Default {
                    }
                    frame 1 {
                    }
                    frame 2 {
                    }
                    frame 3 {
                    }
                    frame 4 {
                    }
                    frame 5 {
                    }
                    frame 6 {
                    }
                  }
                  n193 = call "senPID.vi"("Numeric 3"=w522, "Numeric 2"=w523, "Numeric"=w524, "String"=w525) -> ("String 2"=w527:string)
                  n194 = Wait (ms)(milliseconds to wait=u32 20) -> ()  [unwired: 1 out]
                  n195 = VISA Write(VISA resource name=w521, write buffer=w527, error in (no error)=w520) -> ()  [unwired: 3 out]
                }
              }
              frame 16 {
                n196 = Format Into String(format string="%d", initial string="E", "Min Rang") -> (resulting string=w541:string)  [unwired: 1 in, 1 out]
                n197 = Concatenate Strings(w541, "\n" ("string")) -> (w539:string)
                n198 = VISA Write(VISA resource name=w536, write buffer=w539, error in (no error)=w537) -> ()  [unwired: 3 out]
                n199 = Wait (ms)(milliseconds to wait=u32 10) -> ()  [unwired: 1 out]
              }
              frame 32 {
                n200 = Format Into String(format string="%d", initial string="D", "Max Rang") -> (resulting string=w550:string)  [unwired: 1 in, 1 out]
                n201 = Concatenate Strings(w550, "\n" ("string")) -> (w548:string)
                n202 = VISA Write(VISA resource name=w545, write buffer=w548, error in (no error)=w546) -> ()  [unwired: 3 out]
                n203 = Wait (ms)(milliseconds to wait=u32 10) -> ()  [unwired: 1 out]
              }
              frame 64 {
                n204 = Format Into String(format string="%d", initial string="T", "Turbine Speed") -> (resulting string=w557:string)  [unwired: 1 in, 1 out]
                n205 = Concatenate Strings(w557, "\n" ("string")) -> (w558:string)
                n206 = VISA Write(VISA resource name=w554, write buffer=w558, error in (no error)=w553) -> ()  [unwired: 3 out]
                n207 = Wait (ms)(milliseconds to wait=u32 25) -> ()  [unwired: 1 out]
              }
              frame 128 {
                n208 = Format Into String(format string="%d", initial string="K", 0.0 ("input 1")) -> (resulting string=w566:string)  [unwired: 1 in, 1 out]
                n209 = Concatenate Strings(w566, "\n" ("string")) -> (w567:string)
                n210 = VISA Write(VISA resource name=w564, write buffer=w567, error in (no error)=w563) -> ()  [unwired: 3 out]
                n211 = Wait (ms)(milliseconds to wait=u32 25) -> ()  [unwired: 1 out]
              }
              frame 256 {
                n212 = Format Into String(format string="%d", initial string="W", 0.0 ("input 1")) -> (resulting string=w575:string)  [unwired: 1 in, 1 out]
                n213 = Concatenate Strings(w575, "\n" ("string")) -> (w576:string)
                n214 = VISA Write(VISA resource name=w572, write buffer=w576, error in (no error)=w573) -> ()  [unwired: 3 out]
                n215 = Wait (ms)(milliseconds to wait=u32 25) -> ()  [unwired: 1 out]
              }
              frame 512 {
                n216 = Format Into String(format string="%d", initial string="Y", 0.0 ("input 1")) -> (resulting string=w584:string)  [unwired: 1 in, 1 out]
                n217 = Concatenate Strings(w584, "\n" ("string")) -> (w585:string)
                n218 = VISA Write(VISA resource name=w580, write buffer=w585, error in (no error)=w581) -> ()  [unwired: 3 out]
                n219 = Wait (ms)(milliseconds to wait=u32 25) -> ()  [unwired: 1 out]
              }
            }
          }
        }
      }
    }
  }
  n220 = VISA Close(VISA resource name=w2, error in (no error)=w1) -> ()  [unwired: 1 out]
